vi "NML Multi Chan With Pretrigger.vi"(5 "GAIN & CHANNEL SELECTOR":T2={"0"=3, "1"=4, "2"=0, "3"=0, "4"=0, "5"=0, "6"=0, "7"=0} {"1" scale=0.0..4.0; "0" scale=0.0..4.0; "7" scale=0.0..4.0; "3" scale=0.0..4.0; "5" scale=0.0..4.0; "6" scale=0.0..4.0; "4" scale=0.0..4.0; "2" scale=0.0..4.0}) -> ()   [LabVIEW 2024]
doc: "This VI is designed to scan data from several A/D channels. The first channel is converted to Tesla using the magnet ID (or 'None' for volts). The channels are scanned at an interval of 250µSec/Channel or less.\nScott Hannahs, FBNML, Aug 1992"
uses:
  <vilib>/_DAQmxBase/Internals/DAQmxBase Read (Analog 2D DBL NChan NSamp).vi
  <vilib>/_DAQmxBase/Internals/DAQmxBase Reference Trigger (Analog Edge).vi
panel:
  in  "Trigger Slope":i32(ring)=10280 items=["Rising"=10280, "Falling"=10171]
  out "data":sgl[][](array[numeric]) format="%.3e"
  in  "Trigger Level":sgl(knob) scale=-10.0..10.0 scale format="%.1f"
  in  "time limit (sec)":sgl=5.0 format="%.2f"
  out "timeout?":bool
  in  "?":dbl[](array[numeric])=[1.0, 1.0, 1.0, 1.0, 1.0, 1.0, 1.0, 1.0] format="%.1e"
  in  "Columns Not Plotted":T1
  in  "Comments":string="This data's for you."
  out "?":cluster{dbl[], dbl[]}[](graph)
  in  "Trigger Channel":i16(slide) min=0 max=7 step=1 scale=0.0..7.0
  in  "% Acquired Before Trigger":dbl(knob)=50.0 scale=0.0..100.0
  in  "Column for X-Axis":i32(ring) items=["Point #", "Field", "Column 2", "Column 3", "Column 4", "Column 5", "Column 6", "Column 7", "Column 8", "Column 9", "Column 10"]
  in  "ÆT (msec)":sgl=1.0 min=0 format="%.2f"
  in  "# Points":i32=1000 min=3 max=32000
  out "COLLECTING":bool
  in  "Magnet ID":i32(ring) items=["None", "Cell 12", "Cell 15", "Cell 15insert", "Cell 4", "Cell 4-2", "Cell 4-3", "Cell 5", "Cell 6", "Cell 6-2", "Cell 6-3", "Cell 7", "Cell 8", "Cell 9", "Outsert", "SCM1", "SCM2"]
  out "File Error:":string
  in  "New":bool
  out "Calibration Error":string
  in  "User Name":string="Conan the SCIENTIST"
  out "File Name":string
  in  "File":string="Test"
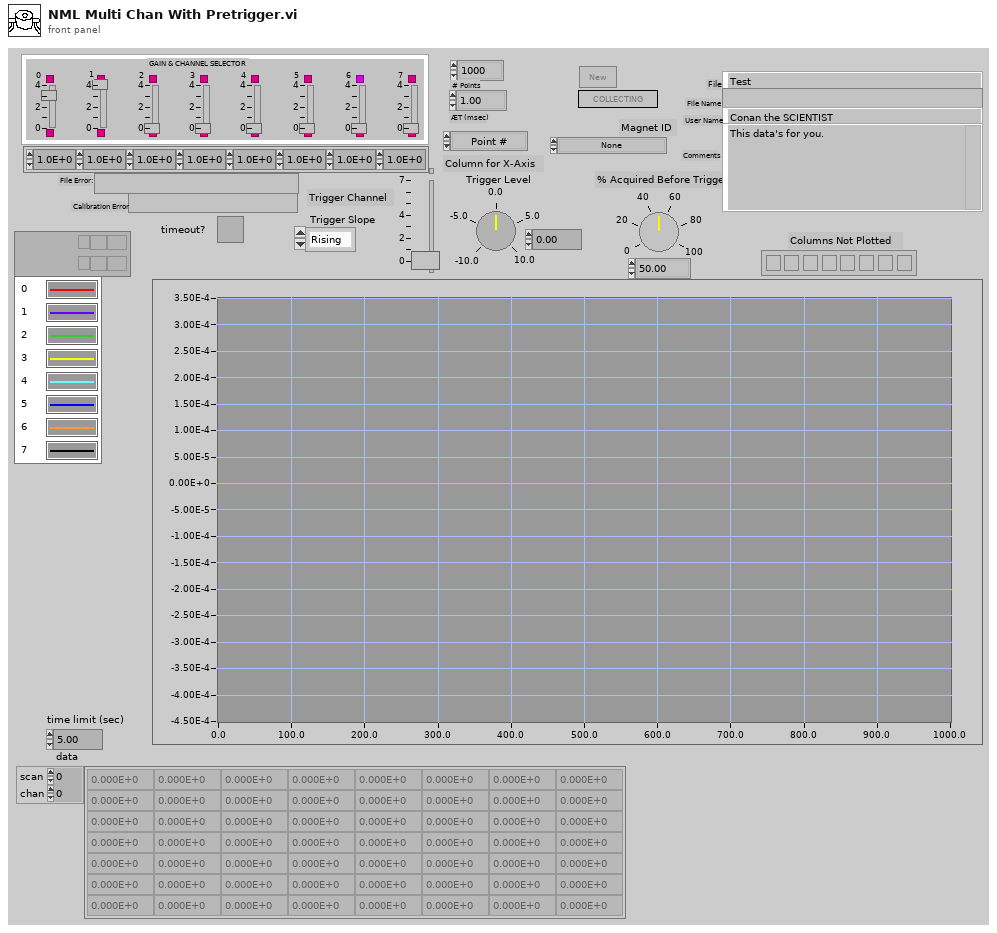
[diagram p1: front panel]
types:
  T1 = cluster{bool, bool, bool, bool, bool, bool, bool, bool}
  T2 = cluster{"0":i16, "1":i16, "2":i16, "3":i16, "4":i16, "5":i16, "6":i16, "7":i16}
  T3 = cluster{"Current Scale Factor kA/V":dbl, "I->B":dbl[], "B->I":dbl[]}
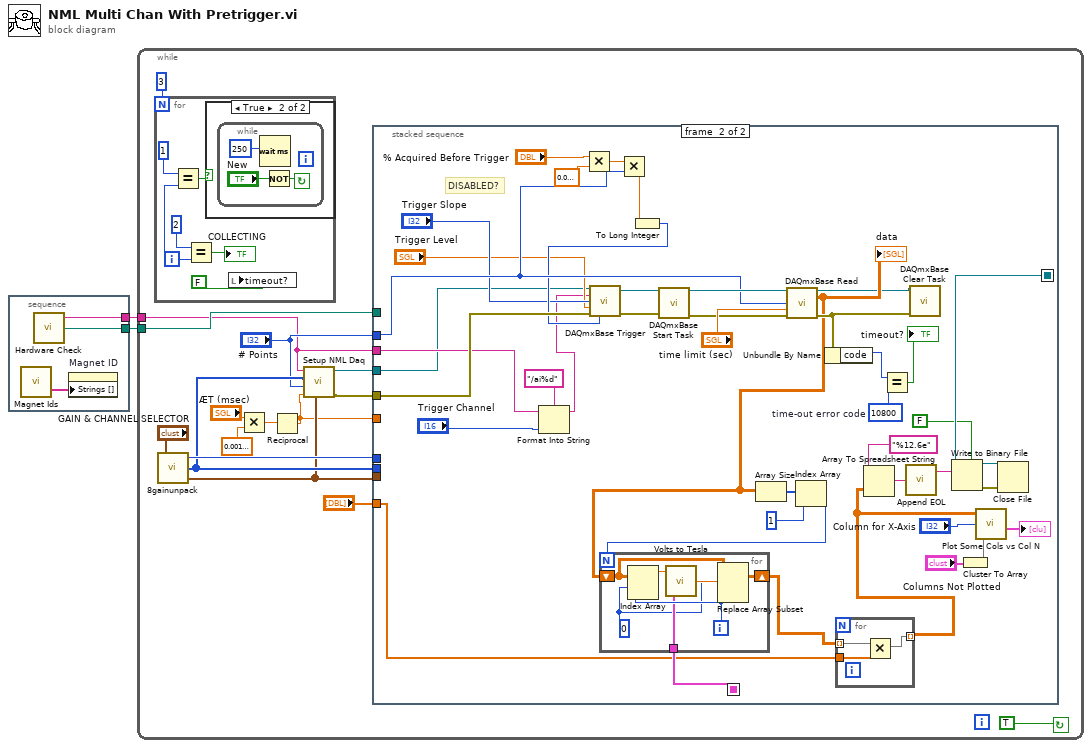
[diagram p0: block diagram]
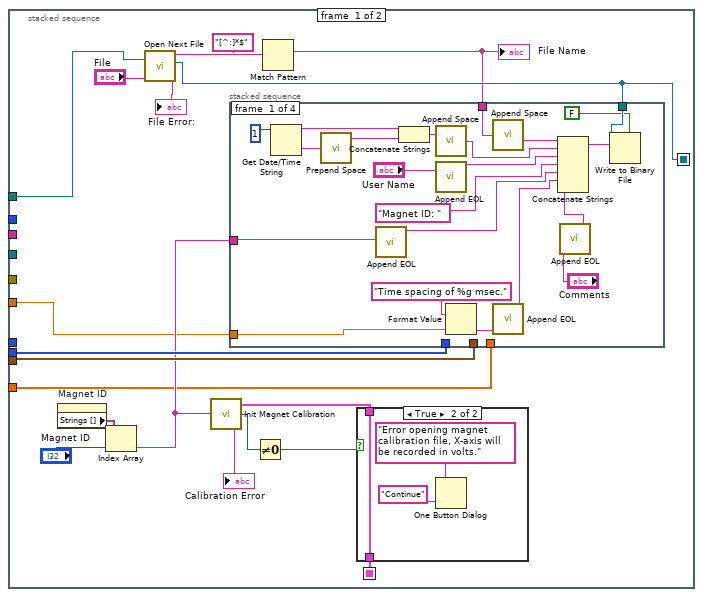
[diagram p3: hidden frame]
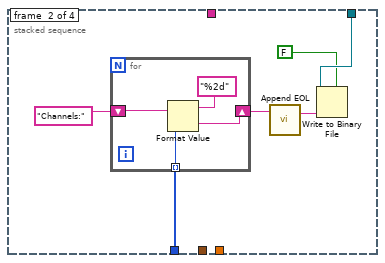
[diagram p5: hidden frame]
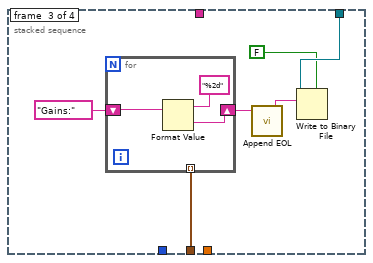
[diagram p6: hidden frame]
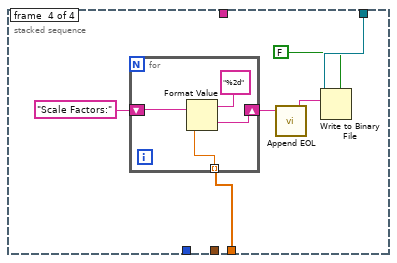
[diagram p7: hidden frame]
diagram:
  n1 = stacked-sequence {
    tunnel: [w4] -> w2
    tunnel: [w3] -> w1
    frame #0 {
      n2 = call "Magnet Ids.vi"() -> ("Magnet IDs"=w5:string[])
      n3 = call "Hardware Check.vi"() -> ("Data Acq Device"=w4:string, "Data Directory Path"=w3:path)  [unwired: 1 in, 1 out]
      n4 = property on="Magnet ID" class="Ring (strict)"("Strings []"=w5) -> ()  [unwired: 2 in, 2 out]
    }
  }
  n5 = while {
    tunnel: w1 -> [w16]
    tunnel: w2 -> [w6]
    stop <- TRUE continue-if-true
    n6 = for {
      N: 3 -> [_]
      i -> [w25]
      n7 = Equal?(x=1, y=w25) -> (x = y?=w24:bool)
      n8 = Equal?(x=2, y=w25) -> (x = y?=→"COLLECTING":bool)
      n9 = case shown="True" w24 {
        frame False {
        }
        frame True {
          n10 = while {
            stop <- w30 continue-if-true
            n11 = Wait (ms)(milliseconds to wait=u32 250) -> ()  [unwired: 1 out]
            n12 = Not(x="New") -> (.not. x?=w30:bool)
          }
        }
      }
      n13 = local write "timeout?"(FALSE) -> ()
    }
    n14 = call "8gainunpack.vi"("GAIN & CHANNEL SELECTOR"="GAIN & CHANNEL SELECTOR") -> ("Number of channels"=w18:i32, "channels (0)"=w13:i32[], "Input Limits"=w8:cluster{"High Limit":dbl, "Low Limit":dbl}[])  [unwired: 1 in]
    n15 = Multiply(x="ÆT (msec)", y=sgl 0.001) -> (x*y=w11:sgl)
    n16 = Reciprocal(x=w11) -> (1/x=w7:sgl)
    n17 = call "Setup NML Daq.vi"("Input Limits"=w8, "rate"=w7, "number of samples per channel"="# Points", "channels (0)"=w13, "Data Acq Device"=w6) -> ("error out"=w14:errorcluster, "task out"=w15:refnum<k21>)  [unwired: 5 in]
    n18 = stacked-sequence {
      seq-local: [w40 _] -> [_ w135]
      seq-local: [w47 _] -> [_ w136]
      tunnel: "?" -> [w35 w134]
      tunnel: w18 -> [_ _]
      tunnel: "# Points" -> [_ w116]
      tunnel: w13 -> [w45 _]
      tunnel: w8 -> [w46 _]
      tunnel: w14 -> [_ w125]
      tunnel: w15 -> [_ w105]
      tunnel: w16 -> [w32 _]
      tunnel: w7 -> [w31 _]
      tunnel: w6 -> [_ w109]
      frame #0 {
        n19 = property on="Magnet ID" class="Ring (strict)"() -> ("Strings []"=w33:string[])  [unwired: 2 in, 2 out]
        n20 = Index Array(array=w33, index="Magnet ID") -> (element=w36:string)
        n21 = call "Open Next File.vi"("Input File Pattern"="File", "Dir Path"=w32) -> ("Error Message"=→"File Error:":string, "File Ref Num"=w47:refnum<file>, "Output File Name"=w49:string)  [unwired: 1 in, 1 out]
        n22 = call "Init Magnet Calibration.vi"("Magnet Id"=w36) -> ("Calibration"=w41:T3, "Error Code"=w42:i32, "Error message"=→"Calibration Error":string)
        n23 = Not Equal To 0?(x=w42) -> (x != 0?=w44:bool)
        n24 = Match Pattern(string=w49, regular expression="[^:]*$") -> (match substring=w39:string)  [unwired: 1 in, 3 out]
        "File Name" <- w39
        n25 = stacked-sequence {
          tunnel: w35 -> [_ _ _ w97]
          tunnel: w31 -> [w57 _ _ _]
          tunnel: w47 -> [w55 w77 w87 w96]
          tunnel: w45 -> [_ w78 _ _]
          tunnel: w46 -> [_ _ w89 _]
          tunnel: w36 -> [w69 _ _ _]
          tunnel: w39 -> [w70 _ _ _]
          frame #0 {
            n26 = Get Date/Time String(date format (0)=1) -> (date string=w61:string, time string=w59:string)  [unwired: 2 in]
            n27 = call "Prepend Space.vi"("Input String"=w59) -> ("Space + Input String"=w60:string)
            n28 = call "Append EOL.vi"("INPUT STRING"=w69) -> ("OUTPUT STRING (PLUS End of Line)"=w64:string)
            n29 = Concatenate Strings(w61, w60) -> (w62:string)
            n30 = call "Append Space.vi"("INPUT STRING"=w62) -> ("OUTPUT STRING (PLUS [SPACE])"=w67:string)
            n31 = call "Append EOL.vi"("INPUT STRING"="User Name") -> ("OUTPUT STRING (PLUS End of Line)"=w66:string)
            n32 = Format Value(format string="Time spacing of %g msec.", value (0)=w57) -> (output string=w72:string)  [unwired: 1 in]
            n33 = call "Append Space.vi"("INPUT STRING"=w70) -> ("OUTPUT STRING (PLUS [SPACE])"=w68:string)
            n34 = call "Append EOL.vi"("INPUT STRING"=w72) -> ("OUTPUT STRING (PLUS End of Line)"=w56:string)
            n35 = call "Append EOL.vi"("INPUT STRING"="Comments") -> ("OUTPUT STRING (PLUS End of Line)"=w63:string)
            n36 = Concatenate Strings(w68, w67, w66, "Magnet ID: ", w64, w56, w63) -> (w75:string)
            n37 = Write to Binary File(file (use dialog)=w55, data=w75, 5:FALSE ("prepend array or string size? (T)")) -> ()  [unwired: 3 in, 3 out]
          }
          frame #1 {
            n38 = for {
              shift-right: [w85] -> w81
              shift-left: "Channels:" -> [w83]
              tunnel: w78 -> [w82] mode=indexing
              n39 = Format Value(string ("")=w83, format string="%2d", value (0)=w82) -> (output string=w85:string)
            }
            n40 = call "Append EOL.vi"("INPUT STRING"=w81) -> ("OUTPUT STRING (PLUS End of Line)"=w80:string)
            n41 = Write to Binary File(file (use dialog)=w77, data=w80, 5:FALSE ("prepend array or string size? (T)")) -> ()  [unwired: 3 in, 3 out]
          }
          frame #2 {
            n42 = for {
              shift-right: [w94] -> w90
              shift-left: "Gains:" -> [w92]
              tunnel: w89 -> [_] mode=indexing
              n43 = Format Value(string ("")=w92, format string="%2d") -> (output string=w94:string)  [unwired: 1 in]
            }
            n44 = call "Append EOL.vi"("INPUT STRING"=w90) -> ("OUTPUT STRING (PLUS End of Line)"=w91:string)
            n45 = Write to Binary File(file (use dialog)=w87, data=w91, 5:FALSE ("prepend array or string size? (T)")) -> ()  [unwired: 3 in, 3 out]
          }
          frame #3 {
            n46 = for {
              shift-right: [w103] -> w99
              shift-left: "Scale Factors:" -> [w101]
              tunnel: w97 -> [w104] mode=indexing
              n47 = Format Value(string ("")=w101, format string="%2d", value (0)=w104) -> (output string=w103:string)
            }
            n48 = call "Append EOL.vi"("INPUT STRING"=w99) -> ("OUTPUT STRING (PLUS End of Line)"=w100:string)
            n49 = Write to Binary File(file (use dialog)=w96, data=w100, 5:FALSE ("prepend array or string size? (T)")) -> ()  [unwired: 3 in, 3 out]
          }
        }
        n50 = case shown="True" w44 {
          tunnel: w41 -> [w50 w51]
          tunnel: [w50 w51] -> w40
          frame False {
          }
          frame True {
            n51 = One Button Dialog(message="Error opening magnet calibration file, X-axis will be recorded in volts.", button name ("OK")="Continue") -> ()  [unwired: 1 out]
          }
        }
      }
      frame #1 {
        w131 = 10800  # time-out error code
        # "DISABLED?"
        # "Magnet Calibration Coefficents"
        n52 = Format Into String(format string="/ai%d", initial string=w109, "Trigger Channel") -> (resulting string=w107:string)  [unwired: 1 in, 1 out]
        n53 = Multiply(x="% Acquired Before Trigger", y=0.009999999776482582) -> (x*y=w124:dbl)
        n54 = Multiply(x=w124, y=w116) -> (x*y=w122:dbl)
        n55 = To Long Integer(number=w122) -> (32bit integer=w113:i32)
        n56 = call-poly <vilib>:"DAQmxBase Trigger.vi"("task/channels in"=w105, "source"=w107, "slope"="Trigger Slope", "level"="Trigger Level", "error in"=w125, "pretrigger samples per channel"=w113) -> ("task out"=w106:refnum<k21>, "error out"=w115:errorcluster)  [unwired: 8 in]
        n57 = call <vilib>:"DAQmxBase Start Task.vi"("task/channels in"=w106, "error in"=w115) -> ("task out"=w129:refnum<k21>, "error out"=w128:errorcluster)  [unwired: 12 in]
        n58 = call-poly <vilib>:"DAQmxBase Read.vi"("task/channels in"=w129, "number of samples per channel"=w116, "timeout"="time limit (sec)", "error in"=w128) -> ("task out"=w117:refnum<k21>, "data"=w126:dbl[][], "error out"=w127:errorcluster)  [unwired: 9 in]
        "data" <- w126
        n59 = Array Size(array=w126) -> (size(s)=w147:i32[])
        n60 = Index Array(array=w147, index=1) -> (element=w120:i32)
        n61 = for {
          N: w120 -> [_]
          shift-right: [w154] -> w119
          shift-left: w126 -> [w153]
          tunnel: w135 -> [w152]
          i -> [w156]
          w151 = 0
          n62 = Index Array(array=w153, index (row)=w151, index (col)=w156) -> (element=w155:dbl)
          n63 = call "Volts to Tesla.vi"("Calibration"=w152, "Console voltage"=w155) -> ("Field"=w157:dbl)
          n64 = Replace Array Subset(array=w153, new element=w157, index (row)=w151, index (col)=w156) -> (w154:dbl[][])
        }
        n65 = Unbundle By Name(w127) -> ("code"=w130:i32)
        n66 = for {
          tunnel: [w148] -> w121 mode=indexing
          tunnel: w119 -> [w149] mode=indexing
          tunnel: w134 -> [w150]
          n67 = Multiply(x=w149, y=w150) -> (x*y=w148:dbl[])
        }
        n68 = Array To Spreadsheet String(array=w121, 3:"%12.6e") -> (spreadsheet string=w139:string)  [unwired: 1 in]
        n69 = Equal?(x=w130, y=w131) -> (x = y?=→"timeout?":bool)
        n70 = call "Append EOL.vi"("INPUT STRING"=w139) -> ("OUTPUT STRING (PLUS End of Line)"=w145:string)
        n71 = call <vilib>:"DAQmxBase Clear Task.vi"("task in"=w117, "error in"=w127) -> ()  [unwired: 13 in, 1 out]
        n72 = Write to Binary File(file (use dialog)=w136, data=w145, 5:FALSE ("prepend array or string size? (T)")) -> (refnum out=w138:refnum<file>, error out=w137:errorcluster)  [unwired: 3 in, 1 out]
        n73 = Cluster To Array(cluster="Columns Not Plotted") -> (array=w140:bool[])
        n74 = call "Plot Some Cols vs Col N.vi"("Display/hide"=w140, "Column for abscissa"="Column for X-Axis", "Input Array"=w121) -> ("Output Graph"=→"?":cluster{dbl[], dbl[]}[])
        n75 = Close File(refnum=w138, error in=w137) -> ()  [unwired: 2 out]
      }
    }
  }
